vi "get_fft_filter.vi"(9 "Modulation info":T1={"Fs full"=0.0, "Fs high"=0.0, "Fs low"=0.0, "Read size"=0, "FFT size low"=5000, "df low"=5000.0, "High carriers"=[], "Low carriers"=[], "Hi channels at low"=[7]} {"Hi channels at low" min=0 step=1; "Low carriers" format="%#_6p"; "High carriers" format="%#_6p"}, 10 "Config":T2={"I/O"={"Buffering (in/out)"=[1.9, 6.0], "Output Device"=1, "Sound"={"sample rate (S/s)"=96000.0, "number of channels"=2, "bits per sample"=24}, "Input Device"=4}, "Noise limit low"=101.5, "Distortion LF cut"=101.5, "Averaging Tc"=3.0, "High rate STFT"={"Win param"=101.5, "Window type"=61, "Win order"=2, "DFT size"=64, "Channels"=[7], "Oversample"=64}, "Low rate STFT"={"Win param"=120.0, "Window type"=61, "Win order"=8, "DFT size"=64, "Channels"=[7], "Oversample"=64}, "Hum filter"={"Frequency"=0.0, "Tc"=0.0}} {"Low rate STFT"."Oversample" min=1 step=1; "Low rate STFT"."Channels" min=0 step=1; "Low rate STFT"."DFT size" min=1 step=1; "Low rate STFT"."Window type" items=["Rectangle"=0, "Hanning"=1, "Hamming"=2, "Blackman-Harris"=3, "Exact Blackman"=4, "Blackman"=5, "Flat Top"=6, "4 Term B-Harris "=7, "7 Term B-Harris"=8, "Low Sidelobe"=9, "Blackman Nuttall"=11, "Triangle"=30, "Bartlett-Hanning"=31, "Bohman"=32, "Parzen"=33, "Welch"=34, "Kaiser"=60, "Dolph-Chebyshev"=61, "Gaussian"=62]; "High rate STFT"."Oversample" min=1 step=1; "High rate STFT"."Channels" min=0 step=1; "High rate STFT"."DFT size" min=1 step=1; "High rate STFT"."Window type" items=["Rectangle"=0, "Hanning"=1, "Hamming"=2, "Blackman-Harris"=3, "Exact Blackman"=4, "Blackman"=5, "Flat Top"=6, "4 Term B-Harris "=7, "7 Term B-Harris"=8, "Low Sidelobe"=9, "Blackman Nuttall"=11, "Triangle"=30, "Bartlett-Hanning"=31, "Bohman"=32, "Parzen"=33, "Welch"=34, "Kaiser"=60, "Dolph-Chebyshev"=61, "Gaussian"=62]; "I/O"."Input Device" format="%.0x"; "I/O"."Output Device" format="%.0x"}, 11 "Averaged FFT":cdb[](array[numeric])) -> (2 "Carrier model":cdb[](array[numeric]), 3 "Distortion filter":cdb[](array[numeric]))   [LabVIEW 2014]
uses:
  ilemt_config.ctl
  <vilib>/sound2/lvsound2.llb/Sound Data Format.ctl
  stft_params.ctl
  <vilib>/Analysis/4window.llb/windowTd.ctl
  modulation_info.ctl
  <vilib>/Analysis/NI_AALPro.lvlib
panel:
  # "Take FFT and separatelthe stuff that is supposed to be there (the carriers) and the stuff that isn't (distortion).   Other stuff like hum isn't phase coherent and gets attenuated in the averaged FFT."
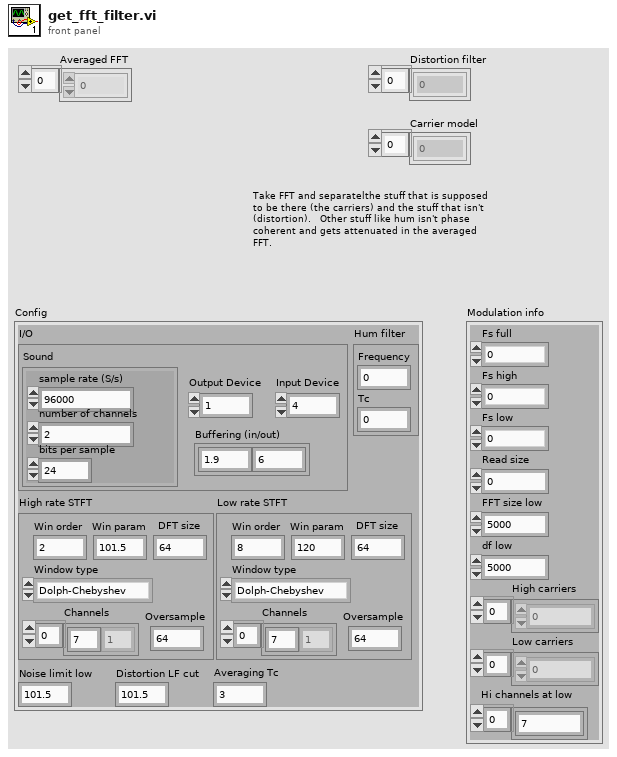
[diagram p1: front panel]
types:
  T1 = typedef "modulation_info.ctl" = cluster{"Fs full":dbl, "Fs high":dbl, "Fs low":dbl, "Read size":i32, "FFT size low":i32, "df low":dbl, "High carriers":dbl[], "Low carriers":dbl[], "Hi channels at low":i32[]}
  T2 = typedef "ilemt_config.ctl" = cluster{"I/O":cluster{"Buffering (in/out)":dbl[], "Output Device":u32, "Sound":T3, "Input Device":u32}, "Noise limit low":dbl, "Distortion LF cut":dbl, "Averaging Tc":sgl, "High rate STFT":T4, "Low rate STFT":T4, "Hum filter":cluster{"Frequency":dbl, "Tc":dbl}}
  T3 = typedef "Sound Data Format.ctl" = cluster{"sample rate (S/s)":dbl, "number of channels":i32, "bits per sample":i32}
  T4 = typedef "stft_params.ctl" = cluster{"Win param":dbl, "Window type":T5, "Win order":i32, "DFT size":i32, "Channels":i32[], "Oversample":i32}
  T5 = typedef "NI_AALPro.lvlib/windowTd.ctl" = u32
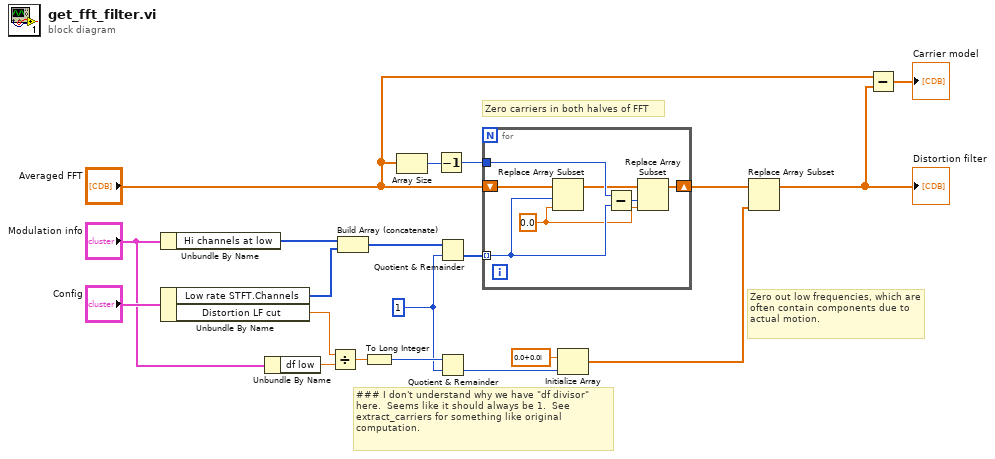
[diagram p0: block diagram]
diagram:
  w1 = 1 ("Low decimate")
  # "### I don't understand why we have \"df divisor\" here.  Seems like it should always be 1.  See extract_carriers for something like original computation."
  # "Zero out low frequencies, which are often contain components due to actual motion."
  # "Zero carriers in both halves of FFT"
  n1 = Unbundle By Name("Modulation info") -> ("Hi channels at low"=w16:i32[])
  n2 = Unbundle By Name("Config") -> ("Low rate STFT.Channels"=w19:i32[], "Distortion LF cut"=w9:dbl)
  n3 = Unbundle By Name("Modulation info") -> ("df low"=w10:dbl)
  n4 = Divide(x=w9, y=w10) -> (x/y=w8:dbl)
  n5 = Build Array (concatenate)(w16, w19) -> (w14:i32[])
  n6 = To Long Integer(number=w8) -> (32bit integer=w7:i32)
  n7 = Array Size(array="Averaged FFT") -> (size(s)=w13:i32)
  n8 = Decrement(x=w13) -> (x-1=w18:i32)
  n9 = Quotient & Remainder(x=w14, y=w1) -> (floor(x/y)=w12:i32[])  [unwired: 1 out]
  n10 = Quotient & Remainder(x=w7, y=w1) -> (floor(x/y)=w6:i32)  [unwired: 1 out]
  n11 = for {
    shift-right: [w22] -> w4
    shift-left: "Averaged FFT" -> [w27]
    tunnel: w12 -> [w25] mode=indexing
    tunnel: w18 -> [w26]
    w21 = 0.0
    n12 = Replace Array Subset(array=w27, new element=w21, index=w25) -> (w23:cdb[])
    n13 = Subtract(x=w26, y=w25) -> (x-y=w24:i32)
    n14 = Replace Array Subset(array=w23, new element=w21, index=w24) -> (w22:cdb[])
  }
  n15 = Initialize Array(cdb 0.0+0.0i, w6) -> (w2:cdb[])
  n16 = Replace Array Subset(array=w4, new element=w2) -> (w3:cdb[])  [unwired: 1 in]
  "Distortion filter" <- w3
  n17 = Subtract(x="Averaged FFT", y=w3) -> (x-y=→"Carrier model":cdb[])
